vi "Investigation LabVIEW Icon.vi"() -> ()   [LabVIEW 2020]
uses:
  C:/Users/Petru/Documents/LabVIEW Data/PopupMenus/edit time panel and diagram/Templates/Target Library/Target Library.lvlib
  <vilib>/LabVIEW Icon API/LabVIEW Icon API.lvlib
  C:/Users/Petru/Documents/LabVIEW Data/PopupMenus/edit time panel and diagram/Templates/Target Library/Owned VI.vi
  <vilib>/LabVIEW Icon API/lv_icon/Classes/Icon/Icon.lvclass
  <vilib>/LabVIEW Icon API/lv_icon/Classes/Layer/Layer.lvclass
  <vilib>/LabVIEW Icon API/lv_icon/Classes/Icon Framework/Icon Framework.lvclass
panel:
  out "VI Icon":refnum<class "Icon.lvclass">
  out "Target Library":refnum<vi>
  # "Investigation LabVIEW Icon"
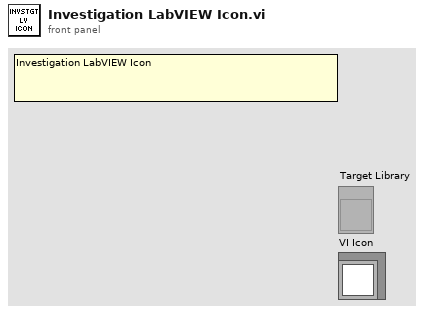
[diagram p1: front panel]
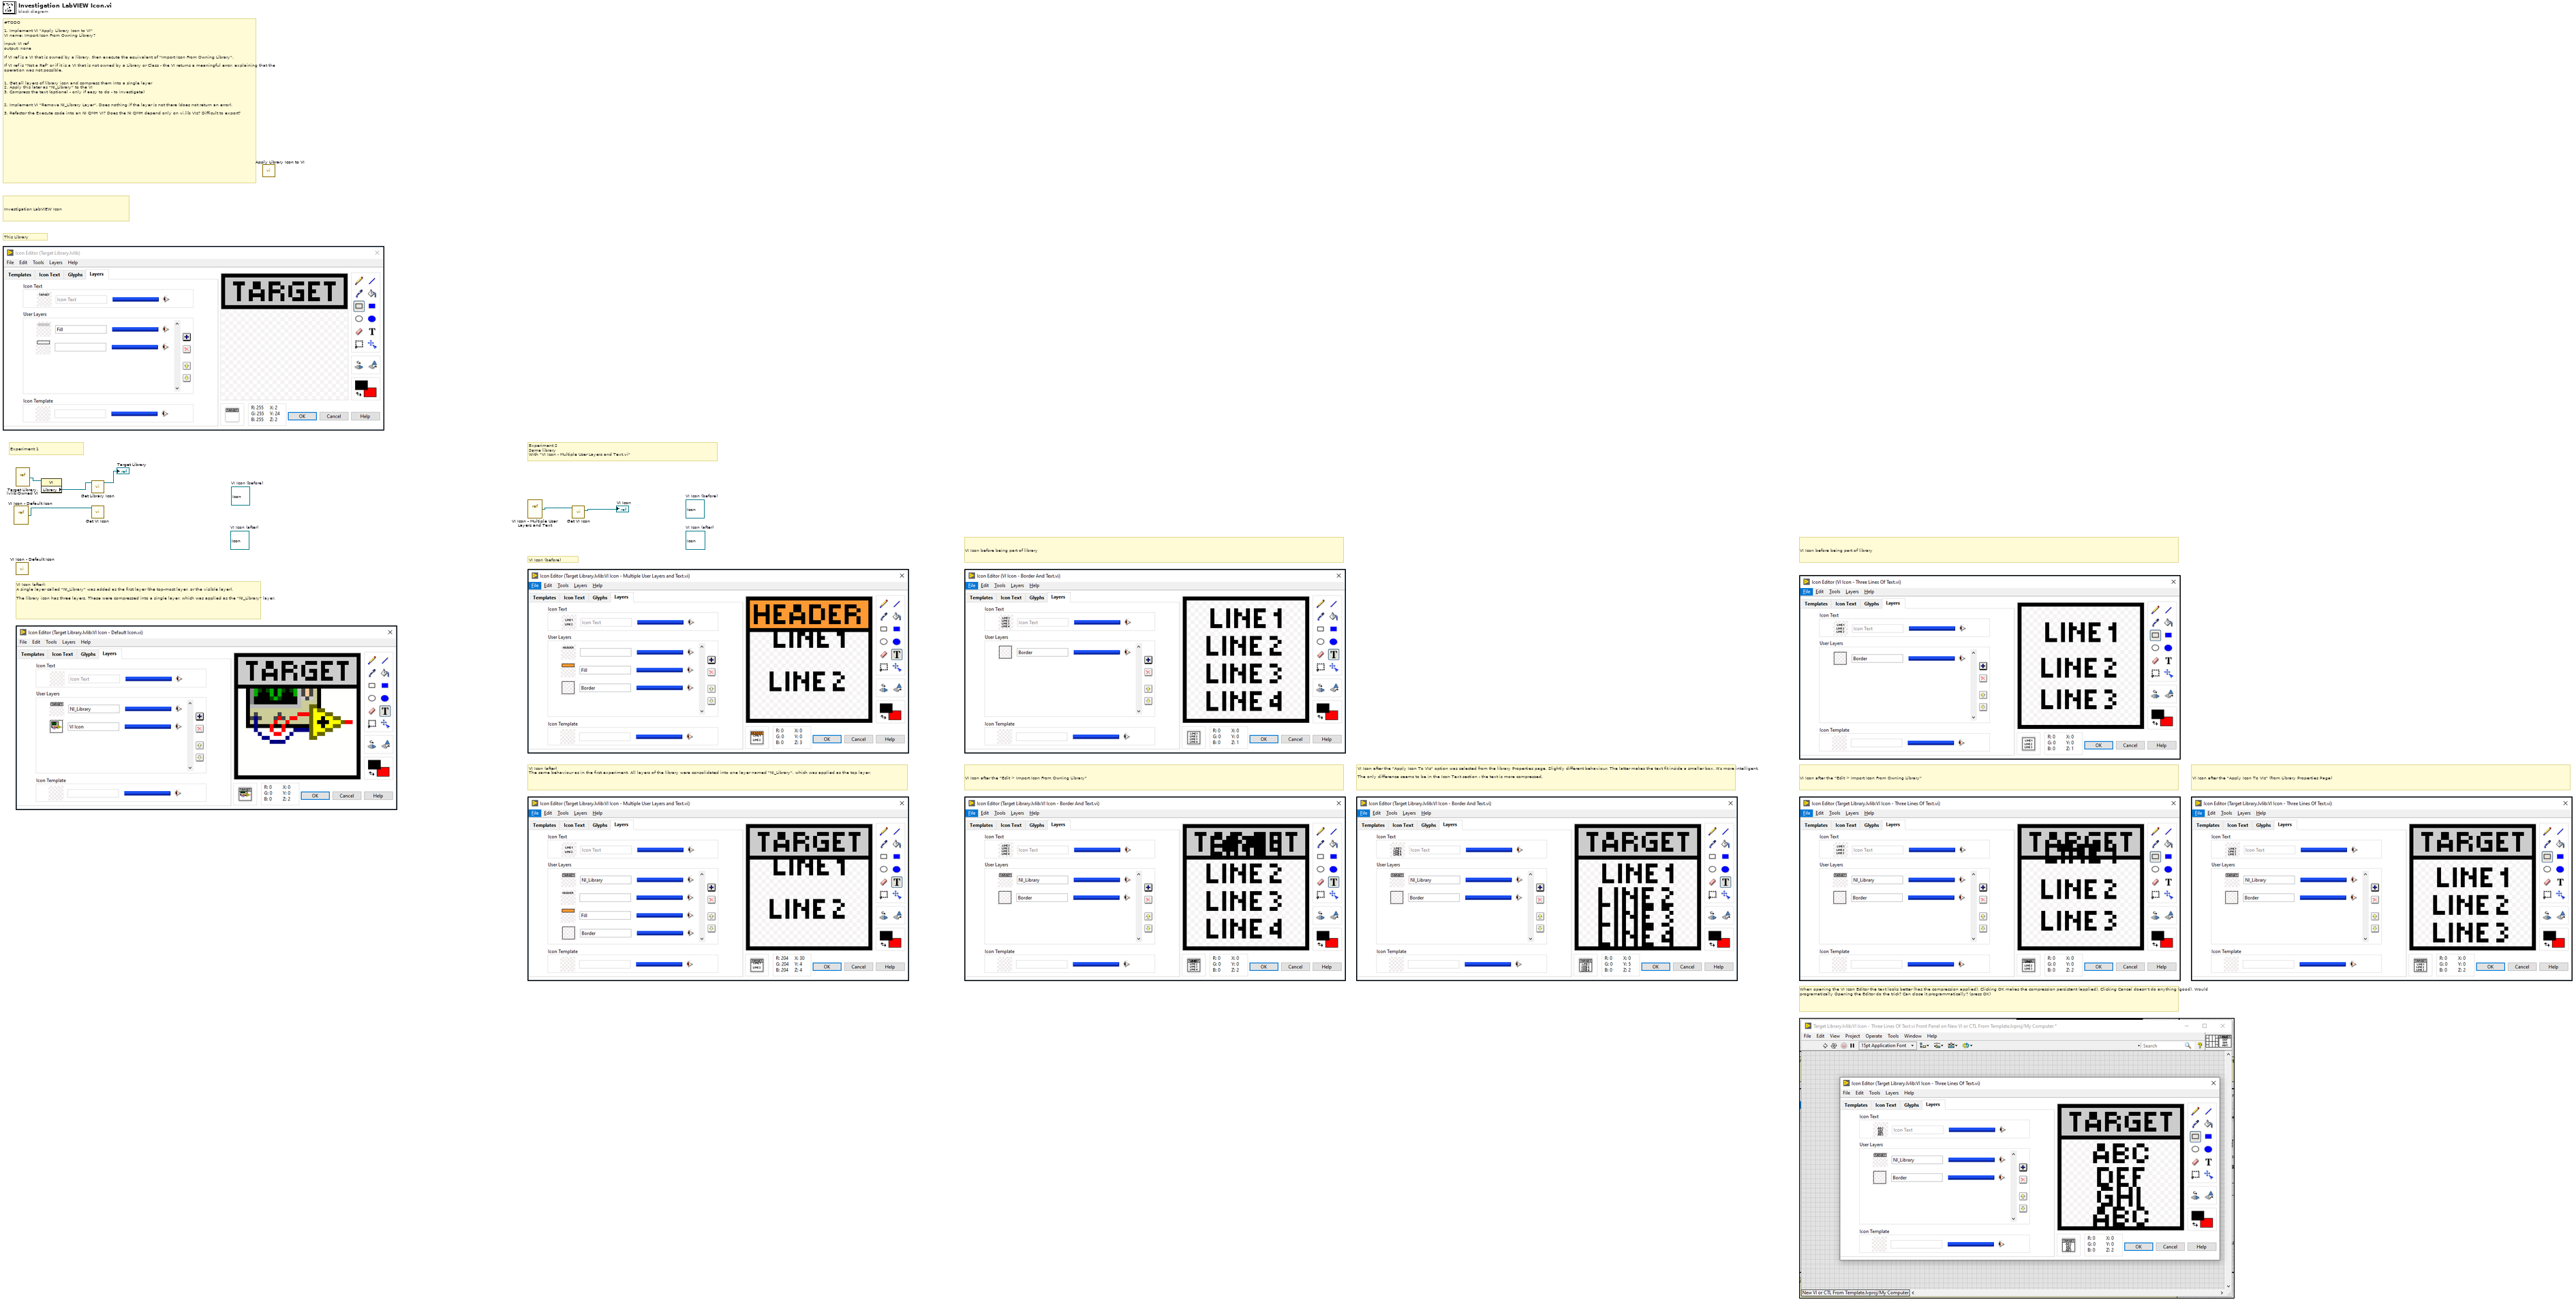
[diagram p0: block diagram]
diagram:
  (unwired) refnum<class "Icon.lvclass"> refnum  # VI Icon (after)
  (unwired) refnum<class "Icon.lvclass"> refnum  # VI Icon (before)
  (unwired) refnum<class "Icon.lvclass"> refnum  # VI Icon (after)
  (unwired) refnum<class "Icon.lvclass"> refnum  # VI Icon (before)
  # "When opening the VI Icon Editor the text looks better (has the compression applied). Clicking OK makes the compression persistent (applied). Clicking Cancel doesn't do anything (good). Would programatically Opening the Editor do the trick? Can close it programmatically? (press OK)"
  # "VI Icon after the \"Apply Icon To VIs\" (from Library Properties Page)"
  # "VI Icon before being part of library"
  # "VI Icon before being part of library"
  # "VI Icon after the \"Edit > Import Icon From Owning Library\""
  # "VI Icon after the \"Apply Icon To VIs\" option was selected from the library Properties page. Slightly different behaviour. The latter makes the text fit inside a smaller box. It's more intelligent.\n\nThe only difference seems to be in the Icon Text section - the text is more compressed."
  # "VI Icon after the \"Edit > Import Icon From Owning Library\""
  # "VI Icon (after)\nThe same behaviour as in the first experiment. All layers of the library were consolidated into one layer named \"NI_Library\", which was applied as the top layer."
  # "VI Icon (before)"
  # "Experiment 2\nSame library\nWith \"VI Icon - Multiple User Layers and Text.vi\""
  # "Experiment 1"
  # "#TODO\n\n1. Implement VI \"Apply Library Icon to VI\"\nVI name: Import Icon From Owning Library?\n\ninput: VI ref\noutput: none\n\nIf VI ref is a VI that is owned by a library, then execute the equivalent of \"Import Icon From Owning Library\".\n\nIf VI ref is \"Not a Ref\" or if it is a VI that is not owned by a Library or Class - the VI returns a meaningful error, explaining that the operation was not possible.\n\n\n1. Get all layers of library icon and compress them into a single layer\n2. Apply this later as \"NI_Library\" to the VI\n3. Compress the text (optional - only if easy to do - to investigate)\n\n\n2. Implement VI \"Remove NI_Library Layer\". Does nothing if the layer is not there (does not return an error).\n\n3. Refactor the Execute code into an NI QMH VI? Does the NI QMH depend only on vi.lib VIs? Difficult to export?"
  # "VI Icon (after):\nA single layer called \"NI_Library\" was added as the first layer (the top-most layer, or the visible layer).\n\nThe library icon has three layers. These were compressed into a single layer, which was applied as the \"NI_Library\" layer."
  # "This Library"
  # "Investigation LabVIEW Icon"
  n1 = vi-ref "VI Icon - Default Icon.vi"() -> (w3:refnum<vi>)
  n2 = vi-ref "Target Library.lvlib:Owned VI.vi"() -> (w6:refnum<vi>)
  n3 = call "VI Icon - Default Icon.vi"() -> ()  [unwired: 12 in]
  n4 = property class="VI"(reference=w6) -> ("Library"=w5:refnum<vi>)  [unwired: 1 in, 2 out]
  n5 = call <vilib>:"Get Library Icon.vi"("Library Refnum in"=w5) -> ("Library Refnum out"=→"Target Library":refnum<vi>)  [unwired: 8 in, 2 out]
  n6 = call <vilib>:"Get VI Icon.vi"("VI Refnum in"=w3) -> ()  [unwired: 8 in, 3 out]
  n7 = call "Apply Library Icon to VI.vi"() -> ()  [unwired: 11 in, 1 out]
  n8 = vi-ref "VI Icon - Multiple User Layers and Text.vi"() -> (w2:refnum<vi>)
  n9 = call <vilib>:"Get VI Icon.vi"("VI Refnum in"=w2) -> ("Icon"=→"VI Icon":refnum<class "Icon.lvclass">)  [unwired: 8 in, 2 out]
